vi "Configure Measurement (Channel Power).vi"(0 "VISA resource name":refnum<visa-resource-name>, 5 "Bandwidth Filter Type (0: Gaussian)":i32(ring) items=["Gaussian", "Flattop"], 7 "PSD Unit (0: dBm/Hz)":i32(ring) items=["dBm/Hz", "dBm/MHz"], 9 "Integration  Bandwidth (2E+6 Hz)":dbl=2000000.0, 11 "error in (no error)":errorcluster) -> (4 "VISA resource name out":refnum<visa-resource-name>, 15 "error out":errorcluster)   [LabVIEW 2018, in "Agilent MXA Series.lvlib"]
doc: "Sets the Channel Power measurement parameters."
uses:
  Agilent MXA Series.lvlib
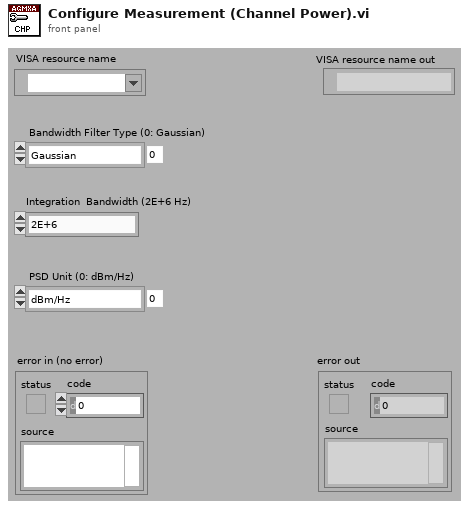
[diagram p1: front panel]
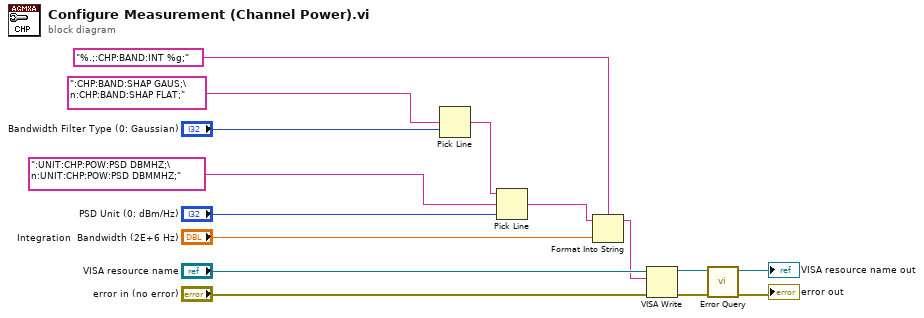
[diagram p0: block diagram]
diagram:
  n1 = Pick Line(multi-line string=":CHP:BAND:SHAP GAUS;\n:CHP:BAND:SHAP FLAT;", line index="Bandwidth Filter Type (0: Gaussian)") -> (output string=w9:string)  [unwired: 1 in]
  n2 = Pick Line(string ("")=w9, multi-line string=":UNIT:CHP:POW:PSD DBMHZ;\n:UNIT:CHP:POW:PSD DBMMHZ;", line index="PSD Unit (0: dBm/Hz)") -> (output string=w8:string)
  n3 = Format Into String(format string="%.;:CHP:BAND:INT %g;", initial string=w8, "Integration  Bandwidth (2E+6 Hz)") -> (resulting string=w1:string)  [unwired: 1 in, 1 out]
  n4 = VISA Write(VISA resource name="VISA resource name", write buffer=w1, error in (no error)="error in (no error)") -> (VISA resource name out=w4:refnum<visa-resource-name>, error out=w5:errorcluster)  [unwired: 1 out]
  n5 = call "Error Query.vi"("error in (no error)"=w5, "VISA resource name"=w4) -> ("error out"=→"error out":errorcluster, "VISA resource name out"=→"VISA resource name out":refnum<visa-resource-name>)  [unwired: 6 in, 2 out]
